vi "clear channel physical units.vi"(6 "Index":u32) -> ()   [LabVIEW 2012]
uses:
  global scale array.vi
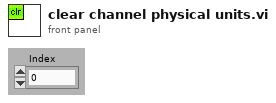
[diagram p1: front panel]
types:
  T1 = typedef "calib array.ctl" = T2[]
  T2 = typedef "conversion.ctl" = cluster{"conversion matrix":sgl[][], "units":string, "name":string, "scale type":T3, "offset (volts)":dbl, "second channel":i8, "correspondence table":T4, "offset (physical units)":dbl, "pH scale":T5, "D.O.":T6}
  T3 = typedef "scale type.ctl" = enum16{"Volts", "Polynomial", "Correspondence Table", "pH", "Dissolved Oxygen", "Quadratic"}
  T4 = typedef "correspondence table.ctl" = cluster{"physical units":dbl, "volts":dbl}[]
  T5 = typedef "pH scale.ctl" = cluster{"Buffers":cluster{"Buffer":dbl, "Calibrated":bool, "V/T":dbl}[], "Temperature":dbl}
  T6 = typedef "DO scale.ctl" = cluster{"Temperature":dbl, "K":dbl, "barometric pressure":dbl}
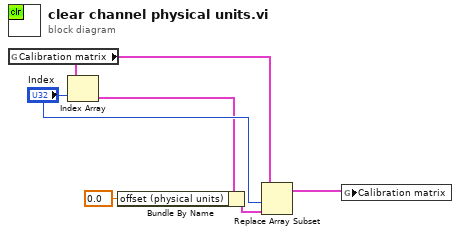
[diagram p0: block diagram]
diagram:
  n1 = global read "global scale array.vi" "Calibration matrix"() -> (w5:T1)
  n2 = Index Array(array=w5, index="Index") -> (element=w2:T2)
  n3 = Bundle By Name(cluster=w2, "offset (physical units)"=0.0) -> (w3:T2)
  n4 = Replace Array Subset(array=w5, new element=w3, index="Index") -> (w4:T1)
  n5 = global write "global scale array.vi" "Calibration matrix"(w4) -> ()
